vi "PRESSURE_CAL.vi"(9 "sim_low":dbl format="%.2f", 10 "sim_high":dbl=1.0 format="%.2f", 11 "Prompt_IN":string) -> (3 "PRESSURE\nFt of water":dbl format="%.2f")   [LabVIEW 2016]
uses:
  ad interface/Global_SIM_switch.vi
panel:
  out "Setup_instructions":string
  in  "OK Button":bool
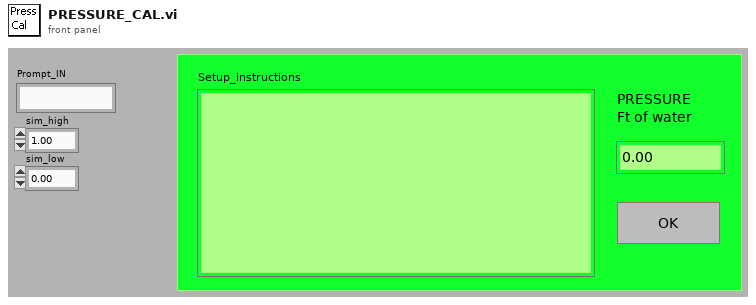
[diagram p1: front panel]
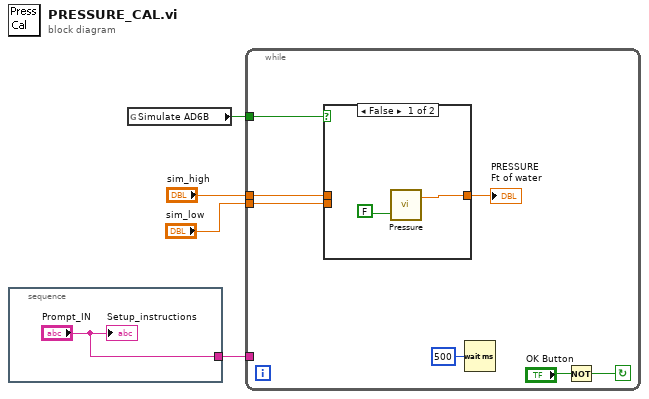
[diagram p0: block diagram]
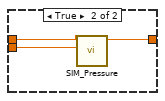
[diagram p2: hidden frame]
diagram:
  n1 = stacked-sequence {
    tunnel: ["Prompt_IN"] -> w3
    frame #0 {
      "Setup_instructions" <- "Prompt_IN"
    }
  }
  n2 = global read "Global_SIM_switch.vi" "Simulate AD6B"() -> (w4:bool)
  n3 = while {
    tunnel: "sim_low" -> [w6]
    tunnel: "sim_high" -> [w7]
    tunnel: w3 -> [_]
    tunnel: w4 -> [w12]
    stop <- w9 continue-if-true
    n4 = case shown="False" w12 {
      tunnel: [w14 w17] -> w11
      tunnel: w7 -> [_ w16]
      tunnel: w6 -> [_ w15]
      frame False {
        n5 = call "Pressure.vi"("Zero Pressure\n(F = leave as is)"=FALSE ("Zero Pressure\n(F = leave as is)")) -> ("Pressure"=w14:dbl)  [unwired: 2 in]
      }
      frame True {
        n6 = call "SIM_Pressure.vi"("sim_low"=w15, "sim_high"=w16) -> ("Pressure"=w17:dbl)  [unwired: 9 in]
      }
    }
    "PRESSURE\nFt of water" <- w11
    n7 = Wait (ms)(milliseconds to wait=u32 500) -> ()  [unwired: 1 out]
    n8 = Not(x="OK Button") -> (.not. x?=w9:bool)
  }
